vi "XNET LIN Schedule Property Node.vi"   [LabVIEW 2018]
doc: "Property node used to read/write properties for an XNET LIN Schedule I/O name."
uses:
  <resource>/objmgr/xnet.rc
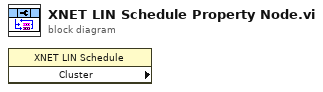
[diagram p0: block diagram]
diagram:
  n1 = property class="XNET LIN Schedule" props=["Cluster"]() -> ()  [unwired: 2 in, 3 out]
